vi "PolhemusAlignment.vi"() -> ()   [LabVIEW 2009]
uses:
  BaudRateSelector.ctl
  <vilib>/Instr/_visa.llb/VISA Configure Serial Port (Instr).vi
panel:
  in  "Parity":enum16{"None", "Odd", "Even", "Mark", "Space"}(ring)
  in  "Data Bits":u16=8 min=7 max=8 step=1
  in  "Baud Rate":T1=115200 items=["1200"=1200, "2400"=2400, "4800"=4800, "9600"=9600, "19200"=19200, "38400"=38400, "57600"=57600, "115200"=115200]
  in  "VISA resource name":refnum<visa-resource-name>="COM3"
  # "Basic Serial Information"
  # "If Data Bits = 8, Parity must be \"None\""
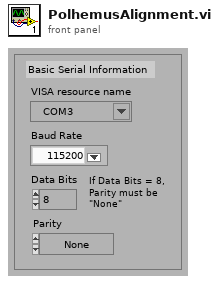
[diagram p1: front panel]
types:
  T1 = typedef "BaudRateSelector.ctl" = u32
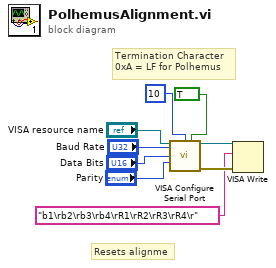
[diagram p0: block diagram]
diagram:
  # "Resets alignme"
  # "Termination Character\n0xA = LF for Polhemus"
  n1 = call-poly "VISA Configure Serial Port"("VISA resource name"="VISA resource name", "termination char\n(0xA = '\\n' = LF)"=u8 10 ("termination char\n(0xA = '\\n' = LF)"), "Enable Termination\nChar (T)"=TRUE ("Enable Termination\nChar (T)"), "baud rate (9600)"="Baud Rate", "data bits (8)"="Data Bits", "parity (0:none)"="Parity") -> ("VISA resource name out"=w2:refnum<visa-resource-name>, "error out"=w3:errorcluster)  [unwired: 8 in]
  n2 = VISA Write(VISA resource name=w2, write buffer="b1\rb2\rb3\rb4\rR1\rR2\rR3\rR4\r", error in (no error)=w3) -> ()  [unwired: 3 out]
